vi "识别训练.vi"() -> ()   [LabVIEW 2018]
uses:
  <vilib>/vision/NI_Vision_Development_Module.lvlib
panel:
  out "String (OCR/OCV 1)":string
  out "error out":errorcluster
  out "Image Out":T1(plugin-control)
  in  "Parameters (OCR/OCV 1)":T2={"Threshold Data"={"Method"=enum."Uniform", "Looking for"=1, "Color Mode"=0, "Kernel Size"={"Width"=32, "Height"=32}, "Ranges"=[{"Min"=1, "Max"=255}]}, "Reject Border"=TRUE, "Number Of Erosions"=0, "Size & Spacing"={"Segment Algorithm"=0, "Min Bounding Rect Width"=1, "Max Bounding Rect Width"=65536, "Min Bounding Rect Height"=1, "Max Bounding Rect Height"=65536, "Min Character Size"=20, "Max Character Size"=65536, "Min Char Spacing"=1, "Max Horiz Element Spacing"=1, "Max Vert Element Spacing"=0, "Max Space Distance"=65536}, "Read Options"={"Read Strategy"=1, "Read Resolution"=2, "Scale Dependant"=FALSE, "Aspect Ratio"=400, "Acceptance Level"=700, "Substitution Character"="?", "MultiLine"=TRUE}, "Valid Characters"=[], "Use Text Pattern"=FALSE, "Orientation"=0, "# Lines Expected"=0, "Number of Blocks"=4} {"Threshold Data"."Looking for" items=["Light on Dark", "Dark on Light"]; "Threshold Data"."Color Mode" items=["RGB", "HSL", "HSV", "HSI"]; "Size & Spacing"."Segment Algorithm" items=["None", "Shortest Segment", "Legacy Auto Split"]; "Read Options"."Read Strategy" items=["Aggressive", "Conservative"]; "Read Options"."Read Resolution" items=["Low", "Medium", "High"]; "Valid Characters"."Pre-defined characters" items=["Any Character", "User-defined Characters", "Alphabetic", "Alphanumeric", "Uppercase Letters", "Lowercase Letters", "Decimal Digits", "Hexadecimal Digits", "Pattern", "Force Space"]; "Orientation" items=["Baseline inside", "Baseline outside"]}
  in  "error in":errorcluster
  in  "退出":bool
  in  "进行识别":bool
  in  "打开文件":bool
types:
  T1 = typedef "IMAQ Image.ctl" = refnum<image>
  T2 = cluster{"Threshold Data":cluster{"Method":enum16{"Fixed Range", "Uniform", "Linear", "Non Linear", "Local", "Color"}, "Looking for":u32, "Color Mode":u32, "Kernel Size":cluster{"Width":i32, "Height":i32}, "Ranges":cluster{"Min":i32, "Max":i32}[]}, "Reject Border":bool, "Number Of Erosions":i32, "Size & Spacing":cluster{"Segment Algorithm":u16, "Min Bounding Rect Width":i32, "Max Bounding Rect Width":i32, "Min Bounding Rect Height":i32, "Max Bounding Rect Height":i32, "Min Character Size":i32, "Max Character Size":i32, "Min Char Spacing":i32, "Max Horiz Element Spacing":i32, "Max Vert Element Spacing":i32, "Max Space Distance":i32}, "Read Options":cluster{"Read Strategy":i32, "Read Resolution":i32, "Scale Dependant":bool, "Aspect Ratio":i32, "Acceptance Level":i32, "Substitution Character":string, "MultiLine":bool}, "Valid Characters":cluster{"Pre-defined characters":i32, "User-defined characters":string}[], "Use Text Pattern":bool, "Orientation":u32, "# Lines Expected":u32, "Number of Blocks":i32}
  T3 = typedef "Image Type" = u32
  T4 = cluster{"Global Rectangle":i32[], "Contours":cluster{"Contour Type":u32, "ROI Type":u32, "Points":i32[]}[]}
  T5 = typedef "IMAQ OCR Session.ctl" = refnum<k1>
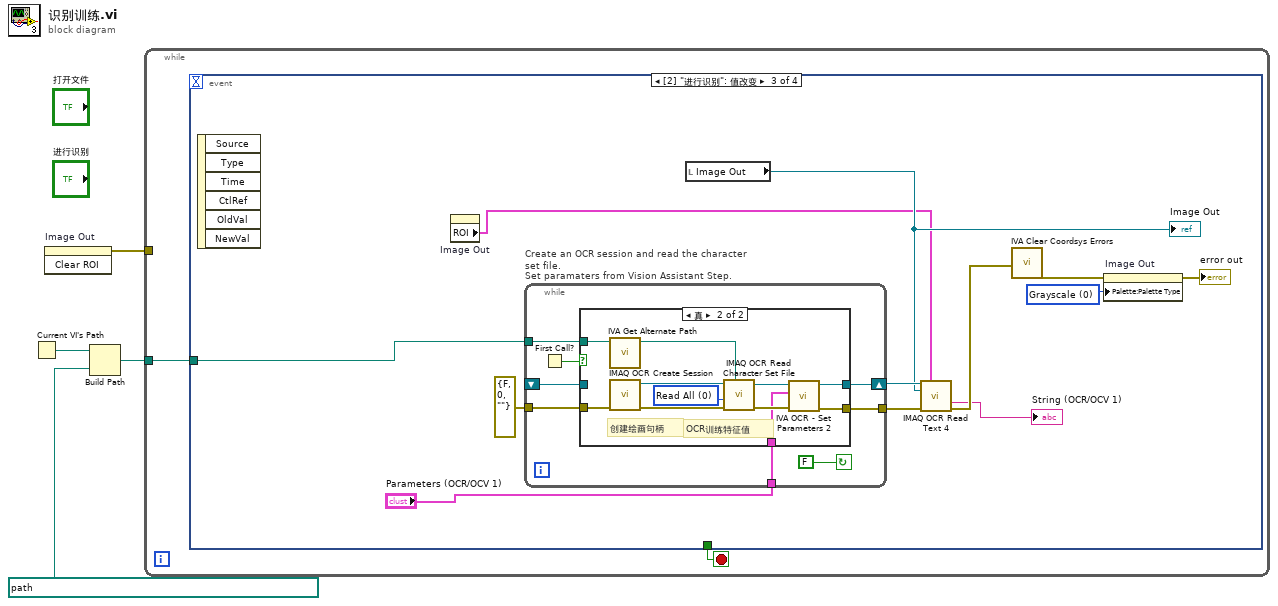
[diagram p0: block diagram]
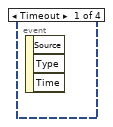
[diagram p2: hidden frame]
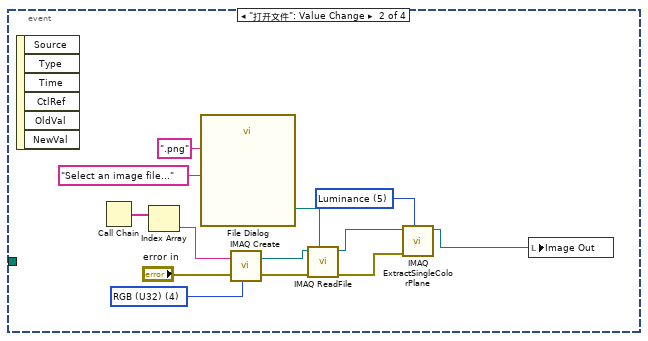
[diagram p3: hidden frame]
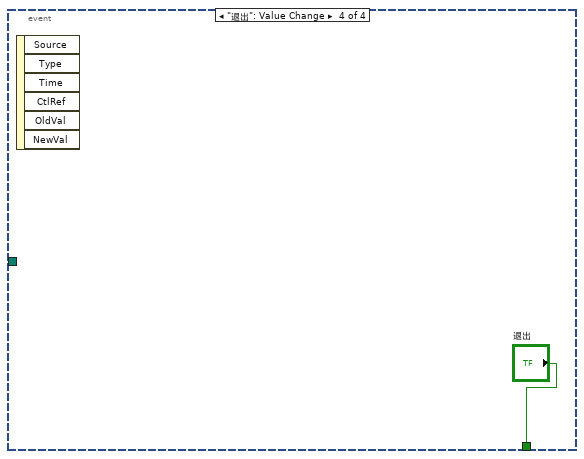
[diagram p5: hidden frame]
diagram:
  n1 = Current VI's Path() -> (path=w3:path)
  n2 = invoke on="Image Out" class="ImageControl" method="Clear ROI"() -> (error out=w1:errorcluster)  [unwired: 3 in, 2 out]
  n3 = Build Path(base path=w3, name or relative path=path "D:/Labviewprogram/视觉/视觉框架/NEW-车牌号.abc" ("路径")) -> (appended path=w4:path)
  n4 = while {
    tunnel: w4 -> [w6]
    tunnel: w1 -> [_]
    stop <- w5 stop-if-true
    n5 = event shown="[2] \"进行识别\": 值改变" {
      selector: _ -> [_ _ _ _]
      dyn-events: _ -> [_ _ _ _]
      timeout: _ -> [_ _ _ _]
      tunnel: w6 -> [_ _ w22 _]
      tunnel: [_ _ _ "退出"] -> w5
      event Timeout {
        n6 = event-data() -> ()  [unwired: 1 in, 3 out]
      }
      event "打开文件": Value Change {
        w8 = 5 items=["Red", "Green", "Blue", "Hue", "Saturation", "Luminance", "Value", "Intensity"] ("Color Plane")
        w19 = T3 4 items=["Grayscale (U8)", "Grayscale (I16)", "Grayscale (SGL)", "Complex (CSG)", "RGB (U32)", "HSL (U32)", "RGB (U64)", "Grayscale (U16)"] ("Image Type")
        n7 = event-data() -> ()  [unwired: 1 in, 6 out]
        n8 = Call Chain() -> (call chain=w15:string[])
        n9 = Index Array(array=w15) -> (element=w16:string)  [unwired: 1 in]
        n10 = call "File Dialog"("prompt"="Select an image file...", "pattern (all files)"=".png") -> ("selected path"=w18:path)  [unwired: 5 in, 8 out]
        n11 = call "IMAQ Create"("Image Name"=w16, "Image Type"=w19, "error in (no error)"="error in") -> ("New Image"=w12:T1, "error out"=w13:errorcluster)  [unwired: 1 in, 1 out]
        n12 = call "IMAQ ReadFile"("File Path"=w18, "error in (no error)"=w13, "Image"=w12) -> ("error out"=w9:errorcluster, "Image Out"=w10:T1)  [unwired: 2 in, 5 out]
        n13 = call "IMAQ ExtractSingleColorPlane"("Color Plane"=w8, "error in (no error)"=w9, "Image Src"=w10) -> ("Image Dst Out"=w7:T1)  [unwired: 7 in, 1 out]
        n14 = local write "Image Out"(w7) -> ()
      }
      event "进行识别": Value Change {
        w31 = u32 0 items=["Grayscale", "Binary", "Gradient", "Rainbow", "Temperature", "User Defined", "Binary 16 Bit", "Gradient 16 Bit", "Rainbow 16 Bit", "Temperature 16 Bit", "User Defined 16 Bit"] ("Palette Type")
        n15 = event-data() -> ()  [unwired: 1 in, 6 out]
        n16 = property on="Image Out" class="ImageControl"() -> ("ROI"=w20:T4)  [unwired: 2 in, 2 out]
        n17 = while "Create an OCR session and read the character set file.\nSet paramaters from Vision Assistant Step." {
          shift-right: [w36] -> w27
          shift-left: _ -> [w35]
          tunnel: errorcluster {"status"=FALSE, "code"=0, "source"=""} ("error out") -> [w38]
          tunnel: "Parameters (OCR/OCV 1)" -> [w34]
          tunnel: w22 -> [w33]
          tunnel: [w32] -> w26
          stop <- FALSE continue-if-true
          n18 = First Call?() -> (First Call?: T/F=w37:bool)
          n19 = case "条件结构" shown="真" w37 {
            tunnel: w33 -> [_ w45]
            tunnel: w38 -> [w40 w49]
            tunnel: [w41 w47] -> w36
            tunnel: [w40 w46] -> w32
            tunnel: w34 -> [_ w42]
            tunnel: w35 -> [w41 _]
            frame False {
            }
            frame True {
              w50 = 0 items=["Read All", "Read Character Set Only", "Read Properties Only"] ("Read Options")
              # "OCR训练特征值"
              # "创建绘画句柄"
              n20 = call <vilib>:"IVA Get Alternate Path.vi"("Path In"=w45) -> ("Path Out"=w44:path)  [unwired: 10 out]
              n21 = call "IMAQ OCR Create Session"("error in (no error)"=w49) -> ("error out"=w51:errorcluster, "IMAQ OCR Session"=w52:T5)  [unwired: 9 out]
              n22 = call "IMAQ OCR Read Character Set File"("File Path"=w44, "error in (no error)"=w51, "Read Options"=w50, "IMAQ OCR Session"=w52) -> ("error out"=w48:errorcluster, "IMAQ OCR Session (dup)"=w43:T5)  [unwired: 1 in, 5 out]
              n23 = call <vilib>:"IVA OCR - Set Parameters 2.vi"("error in (no error)"=w48, "Parameters"=w42, "IMAQ OCR Session"=w43) -> ("error out"=w46:errorcluster, "IMAQ OCR Session Out"=w47:T5)  [unwired: 7 in]
            }
          }
        }
        n24 = local read "Image Out"() -> (w21:T1)
        "Image Out" <- w21
        n25 = call "IMAQ OCR Read Text 4"("IMAQ OCR Session"=w27, "ROI Descriptor"=w20, "Image"=w21, "error in (no error)"=w26) -> ("Read String"=→"String (OCR/OCV 1)":string, "error out"=w28:errorcluster)  [unwired: 2 in, 8 out]
        n26 = call <vilib>:"IVA Clear Coordsys Errors.vi"("error in (no error)"=w28) -> ("error out"=w29:errorcluster)  [unwired: 10 in]
        n27 = property on="Image Out" class="ImageControl"(error in=w29, "Palette:Palette Type"=w31) -> (error out=→"error out":errorcluster)  [unwired: 1 in, 1 out]
      }
      event "退出": Value Change {
        n28 = event-data() -> ()  [unwired: 1 in, 6 out]
      }
    }
  }
